vi "ReadGyro.vi"() -> ()   [LabVIEW 2013]
uses:
  Robot Global Data.vi
panel:
  out "GyroAngle":dbl
  in  "ResetGyro":bool
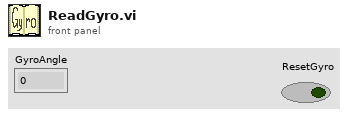
[diagram p1: front panel]
types:
  T1 = typedef "WPI_GyroDevRef.ctl" = cluster{"DevStatus":errorcluster, "Analog Module":T2, "Analog Channel":T3, "Offset":dbl, "Gain (VoltsPerDegree/Second)":dbl}
  T2 = typedef "FPGA_TypedefAnalogModule.ctl" = enum16{"Analog Module 1", "Analog Module 2"}
  T3 = typedef "FPGA_AIChannel.ctl" = enum8{"AI 1", "AI 2", "AI 3", "AI 4", "AI 5", "AI 6", "AI 7", "AI 8", "Invalid"}
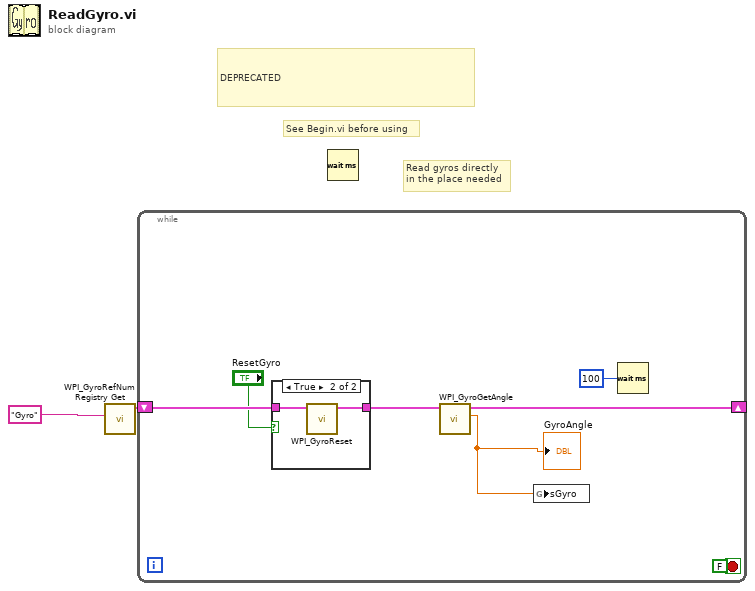
[diagram p0: block diagram]
diagram:
  # "See Begin.vi before using"
  # "DEPRECATED"
  # "Read gyros directly\nin the place needed"
  n1 = call <vilib>:"WPI_GyroRefNum Registry Get.vi"("refnum name"="Gyro") -> ("GyroDevRef"=w1:T1)  [unwired: 9 in, 1 out]
  n2 = while {
    shift-right: [w8] -> _
    shift-left: w1 -> [w7]
    stop <- FALSE stop-if-true
    n3 = case shown="True" "ResetGyro" {
      tunnel: w7 -> [w10 w12]
      tunnel: [w10 w11] -> w4
      frame False {
      }
      frame True {
        n4 = call <vilib>:"WPI_GyroReset.vi"("GyroDevRef"=w12) -> ("GyroDevRef"=w11:T1)  [unwired: 9 in, 1 out]
      }
    }
    n5 = call <vilib>:"WPI_GyroGetAngle.vi"("GyroDevRef"=w4) -> ("Angle"=w3:dbl, "GyroDevRef"=w8:T1)  [unwired: 7 in, 2 out]
    "GyroAngle" <- w3
    n6 = global write "Robot Global Data.vi" "sGyro"(w3) -> ()
    n7 = Wait (ms)(milliseconds to wait=u32 100) -> ()  [unwired: 1 out]
  }
  n8 = Wait (ms)() -> ()  [unwired: 1 in, 1 out]
